vi "Close.vi"(8 "error in":errorcluster, 11 "Config from Excel Table in":refnum<class "Config from Excel Table.lvclass">) -> (0 "error out":errorcluster, 3 "Config from Excel Table out":refnum<class "Config from Excel Table.lvclass">)   [LabVIEW 2025, in "Config from Excel Table.lvclass"]
uses:
  Config from Excel Table.lvclass
  Config from Excel Table.lvclass/Config from Excel Table.ctl
  <vilib>/Peter/Open Xml/Source/Open Xml.lvlib
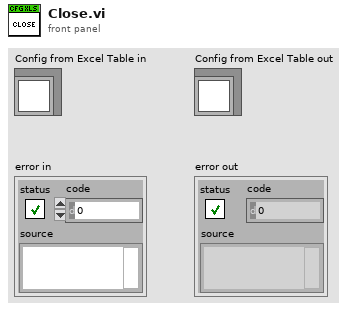
[diagram p1: front panel]
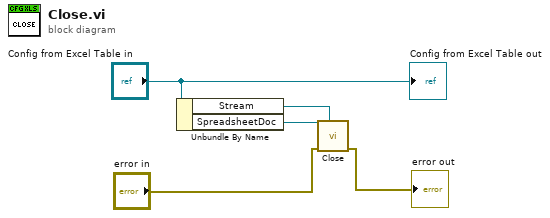
[diagram p0: block diagram]
diagram:
  n1 = Unbundle By Name("Config from Excel Table in") -> ("Stream"=w1:refnum<k24>, "SpreadsheetDoc"=w2:refnum<k24>)
  n2 = call <vilib>:"Close.vi"("Stream"=w1, "error in"="error in", "SpreadsheetDoc"=w2) -> ("error out"=→"error out":errorcluster)  [unwired: 8 in]
  "Config from Excel Table out" <- "Config from Excel Table in"
